vi "8_math_analysis.vi"() -> ()   [LabVIEW 2017]
uses:
  <vilib>/Analysis/NI_AALBase.lvlib
  <vilib>/Analysis/NI_AALPro.lvlib
panel:
  out "Polynomial Coefficients":dbl[](array[numeric])
  out "Waveform Graph":T1(graph)
  in  "polynomial order":i32=2
  out "variance":dbl format="%_2f"
  out "standard deviation":dbl format="%_2f"
  out "mean":dbl format="%_2f"
  out "min index(es)":i32 format="%_2f"
  out "min value":dbl format="%#_2g"
  out "max index(es)":i32 format="%_2f"
  out "max value":dbl format="%#_2g"
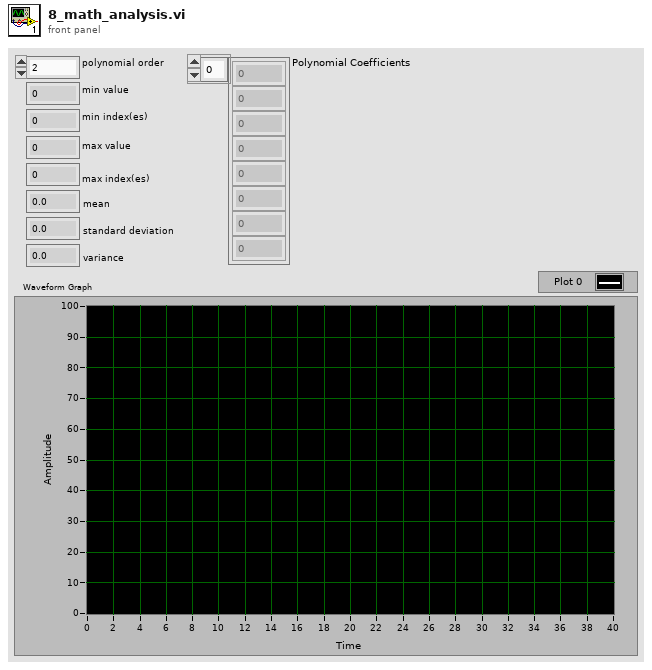
[diagram p1: front panel]
types:
  T1 = cluster{"offset":i32, "frequência":dbl, "Best Polynomial Fit":dbl[]}[]
  T2 = cluster{"offset":i32, "frequência":dbl, "Best Polynomial Fit":dbl[]}
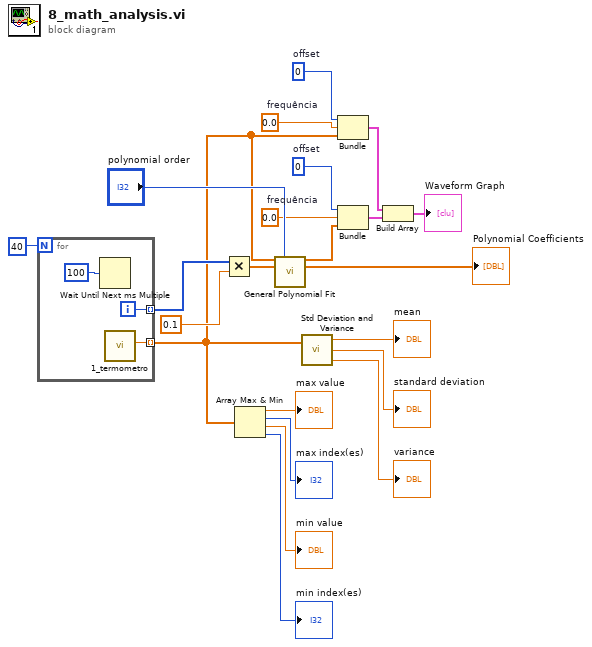
[diagram p0: block diagram]
diagram:
  w6 = 0.0  # frequência
  w7 = 0  # offset
  w9 = 0.0  # frequência
  w10 = 0  # offset
  n1 = for {
    N: 40 -> [_]
    tunnel: [w25] -> w8 mode=indexing
    tunnel: [w23] -> w14 mode=indexing
    i -> [w23]
    n2 = Wait Until Next ms Multiple(millisecond multiple=u32 100) -> ()  [unwired: 1 out]
    n3 = call "1_termometro.vi"() -> ("Celsius"=w25:dbl)  [unwired: 1 in, 3 out]
  }
  n4 = Multiply(x=w14, y=0.1) -> (x*y=w11:dbl[])
  n5 = Array Max & Min(array=w8) -> (max value=→"max value":dbl, max index (indices)=→"max index(es)":i32, min value=→"min value":dbl, min index (indices)=→"min index(es)":i32)
  n6 = call <vilib>:"General Polynomial Fit.vi"("Y"=w8, "polynomial order"="polynomial order", "X"=w11) -> ("Best Polynomial Fit"=w5:dbl[], "Polynomial Coefficients"=→"Polynomial Coefficients":dbl[])  [unwired: 9 in, 2 out]
  n7 = call <vilib>:"Std Deviation and Variance.vi"("X"=w8) -> ("mean"=→"mean":dbl, "standard deviation"=→"standard deviation":dbl, "variance"=→"variance":dbl)  [unwired: 1 in]
  n8 = Bundle("offset"=w10, "frequência"=w9, w8) -> (w4:cluster{"offset":i32, "frequência":dbl, dbl[]})  [unwired: 1 in]
  n9 = Bundle("offset"=w7, "frequência"=w6, "Best Polynomial Fit"=w5) -> (w3:T2)  [unwired: 1 in]
  n10 = Build Array(w4, w3) -> (→"Waveform Graph":T1)
